vi "Init.vi"(1 "Which Index":i32) -> (0 "Action out":refnum<class "Act_Get One.lvclass">)   [LabVIEW 2014, in "Act_Get One.lvclass"]
uses:
  Act_Get One.lvclass
  Act_Get One.lvclass/Act_Get One.ctl
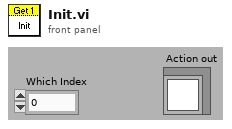
[diagram p1: front panel]
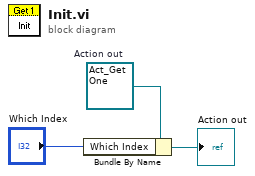
[diagram p0: block diagram]
diagram:
  w3 = refnum<class "Act_Get One.lvclass"> refnum  # Action out
  n1 = Bundle By Name(cluster=w3, "Which Index"="Which Index") -> (→"Action out":refnum<class "Act_Get One.lvclass">)
